vi "go_straight.vi"   [LabVIEW 2013, in "mit2.lvrbt"]
uses:
  mit2.lvrbt
  <vilib>/NXT/Hardware/Plugins/Tetrix DC Motor/TetrixDCMotorAddress.ctl
  <vilib>/NXT/Dual Mode Library/Waits/Wait_Num.vi
  <vilib>/NXT/NXTIO Xnodes/NXTIONodeSubVIs/TETRIX IO Move DC Motors.vi
  <vilib>/NXT/NXTIO Xnodes/NXTIONodeSubVIs/TETRIX IO Stop DC Motors.vi
  <vilib>/NXT/Subs/LVHSConnector.ctl
  <vilib>/NXT/NXTIO Xnodes/AddressXNode/NXTIOAddress.xnode
  <vilib>/NXT/NXTIO Xnodes/NXTIOXNode/NXTIO.xnode
  <vilib>/NXT/LegoClasses/BrickReference/BrickReference.lvclass
types:
  T1 = typedef "TetrixDCMotorAddress.ctl" = i32
  T2 = typedef "LVHSConnector.ctl" = refnum<class "BrickReference.lvclass">
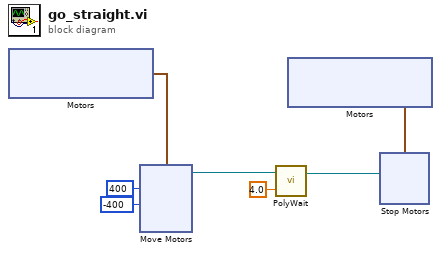
[diagram p0: block diagram]
diagram:
  n1 = xnode "Motors"() -> ("Motor"=w7:cluster{"TetrixDCMotor":T1, "TetrixDCMotor":T1})
  n2 = xnode "Move Motors"("Power/Speed 2"=-400, "Power/Speed 1"=400, "Motors"=w7) -> ("NXT/EV3"=w4:T2)  [unwired: 1 in]
  n3 = call-poly <vilib>:"PolyWait.vi"("Time (1 sec)"=sgl 4.0, "NXT/EV3"=w4) -> ("NXT/EV3"=w2:T2)  [unwired: 2 in]
  n4 = xnode "Motors"() -> ("Motor"=w1:cluster{"TetrixDCMotor":T1, "TetrixDCMotor":T1})
  n5 = xnode "Stop Motors"("Motors"=w1, "NXT/EV3"=w2) -> ()  [unwired: 1 out]
